vi "Set Thread Parameters.vi"(10 "thread settings":T1={"Priority"=100, "Processor"=-2}, 11 "Thread in":refnum<class "Thread.lvclass">) -> (3 "Thread out":refnum<class "Thread.lvclass">)   [LabVIEW 2019, in "DSF Core.lvlib" / "Thread.lvclass"]
uses:
  Thread.lvclass
  Thread Settings.ctl
  Thread.lvclass/Thread.ctl
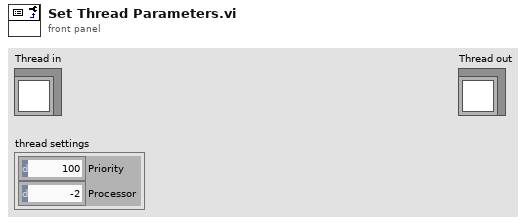
[diagram p1: front panel]
types:
  T1 = typedef "DSF Core.lvlib/Thread.lvclass/Thread Settings.ctl" = cluster{"Priority":u16, "Processor":i32}
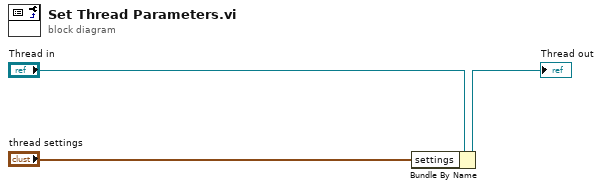
[diagram p0: block diagram]
diagram:
  n1 = Bundle By Name(cluster="Thread in", "settings"="thread settings") -> (→"Thread out":refnum<class "Thread.lvclass">)
